vi "PQgetvalue.vi"(8 "error in (no error)":errorcluster, 9 "column_number":i32, 10 "row_number":i32, 11 "res":u32) -> (0 "error out":errorcluster, 3 "field_value":string)   [LabVIEW 2018, in "libpqlv.lvlib"]
doc: "Returns a single field value of one row of a PGresult. Row and column numbers start at 0. The caller should not free the result directly. It will be freed when the associated PGresult handle is passed to PQclear."
uses:
  libpqlv.lvlib
  lib/libpq.dll
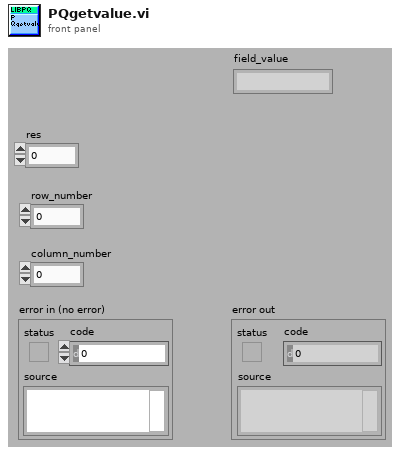
[diagram p1: front panel]
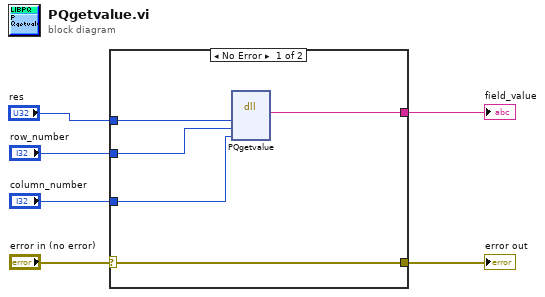
[diagram p0: block diagram]
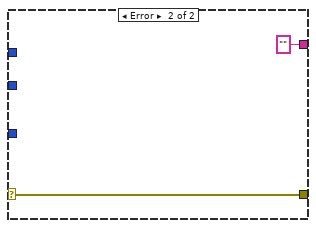
[diagram p2: hidden frame]
diagram:
  n1 = case shown="No Error" "error in (no error)" {
    selector: "error in (no error)" -> [w11 w13]
    tunnel: [w11 w13] -> w5
    tunnel: [w10 "" ("field_value")] -> w4
    tunnel: "row_number" -> [w9 _]
    tunnel: "column_number" -> [w8 _]
    tunnel: "res" -> [w7 _]
    frame No Error {
      n2 = dll-call lib="D:/Users/erics/Documents/TC-3/DAQ/PostgreSQL2LabVIEW/libpqlv/lib/libpq.*" fn="PQgetvalue"("res"=w7, "row_number"=w9, "column_number"=w8) -> ("field_value"=w10:string)  [unwired: 6 in, 2 out]
    }
    frame Error {
    }
  }
  "field_value" <- w4
  "error out" <- w5
